vi "ExSubSetPulserInSpeFileHeader.vi"(3 "error in (no error)":errorcluster, 4 "Pulser Handle":u32, 5 "File Handle":u32) -> (0 "error out":errorcluster, 1 "Pulser Handle":u32, 2 "File Handle":u32)   [LabVIEW 2010]
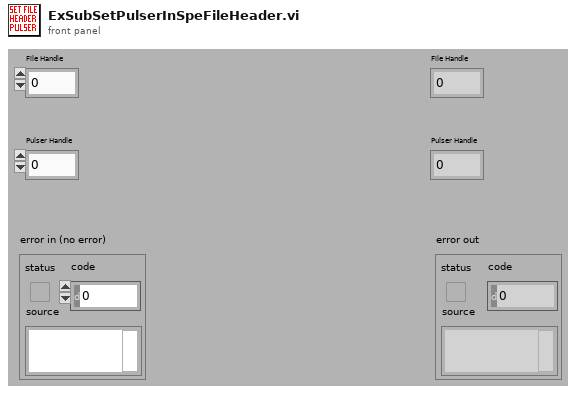
[diagram p1: front panel]
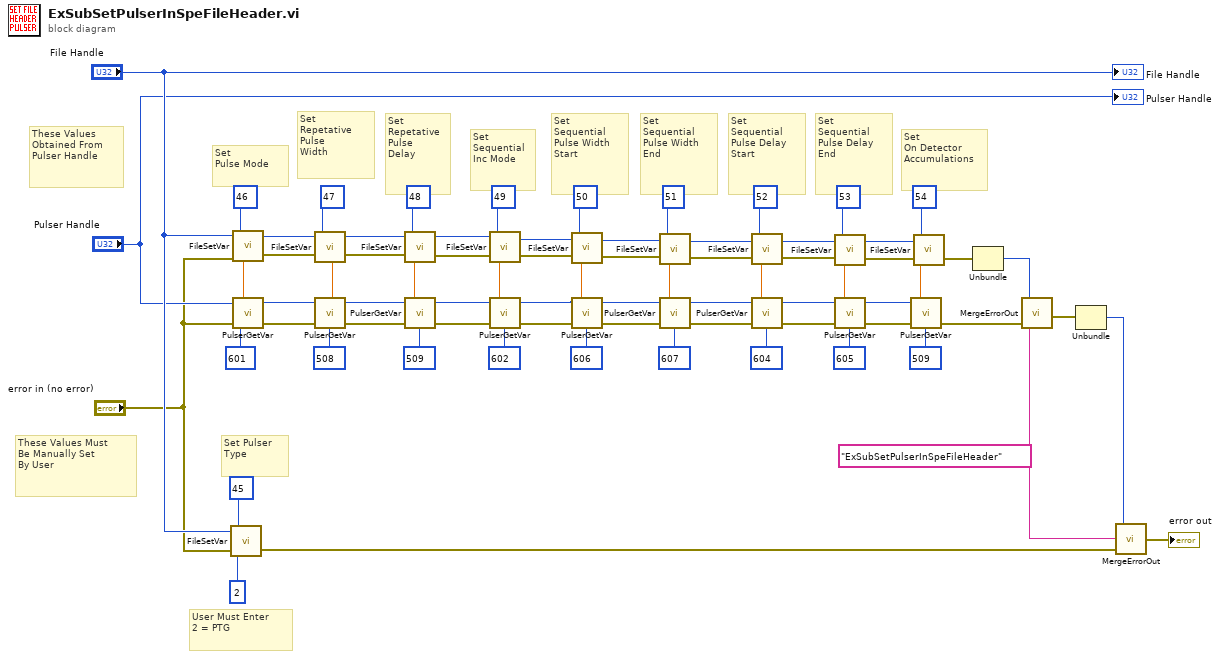
[diagram p0: block diagram]
diagram:
  w7 = "ExSubSetPulserInSpeFileHeader"
  # "These Values Must\nBe Manually Set\nBy User"
  # "These Values\nObtained From\nPulser Handle"
  # "User Must Enter\n2 = PTG"
  # "Set Pulser\nType"
  # "Set \nOn Detector\nAccumulations"
  # "Set\nSequential\nPulse Delay\nEnd"
  # "Set\nSequential\nPulse Delay\nStart"
  # "Set\nSequential\nPulse Width\nEnd"
  # "Set\nSequential\nPulse Width\nStart"
  # "Set\nSequential\nInc Mode"
  # "Set\nRepetative\nPulse\nDelay"
  # "Set\nRepetative\nPulse\nWidth"
  # "Set\nPulse Mode"
  n1 = call <userlib>:"FileSetVar.vi"("error in"="error in (no error)", "Value"=2, "Parameter ID"=45, "File Handle"="File Handle") -> ("error out"=w3:errorcluster)  [unwired: 1 out]
  n2 = call <userlib>:"PulserGetVar.vi"("error in (no error)"="error in (no error)", "Parameter ID"=601, "Pulser Handle"="Pulser Handle") -> ("error out"=w60:errorcluster, "Value"=w70:dbl, "Pulser Handle"=w62:u32)
  n3 = call <userlib>:"FileSetVar.vi"("error in"="error in (no error)", "Value"=w70, "Parameter ID"=46, "File Handle"="File Handle") -> ("error out"=w58:errorcluster, "File Handle"=w67:u32)
  n4 = call <userlib>:"PulserGetVar.vi"("error in (no error)"=w60, "Parameter ID"=508, "Pulser Handle"=w62) -> ("error out"=w59:errorcluster, "Value"=w57:dbl, "Pulser Handle"=w61:u32)
  n5 = call <userlib>:"FileSetVar.vi"("error in"=w58, "Value"=w57, "Parameter ID"=47, "File Handle"=w67) -> ("error out"=w65:errorcluster, "File Handle"=w66:u32)
  n6 = call <userlib>:"PulserGetVar.vi"("error in (no error)"=w59, "Parameter ID"=509, "Pulser Handle"=w61) -> ("error out"=w49:errorcluster, "Value"=w56:dbl, "Pulser Handle"=w50:u32)
  n7 = call <userlib>:"FileSetVar.vi"("error in"=w65, "Value"=w56, "Parameter ID"=48, "File Handle"=w66) -> ("error out"=w51:errorcluster, "File Handle"=w52:u32)
  n8 = call <userlib>:"PulserGetVar.vi"("error in (no error)"=w49, "Parameter ID"=602, "Pulser Handle"=w50) -> ("error out"=w24:errorcluster, "Value"=w53:dbl, "Pulser Handle"=w28:u32)
  n9 = call <userlib>:"FileSetVar.vi"("error in"=w51, "Value"=w53, "Parameter ID"=49, "File Handle"=w52) -> ("error out"=w32:errorcluster, "File Handle"=w36:u32)
  n10 = call <userlib>:"PulserGetVar.vi"("error in (no error)"=w24, "Parameter ID"=606, "Pulser Handle"=w28) -> ("error out"=w23:errorcluster, "Value"=w46:dbl, "Pulser Handle"=w27:u32)
  n11 = call <userlib>:"FileSetVar.vi"("error in"=w32, "Value"=w46, "Parameter ID"=50, "File Handle"=w36) -> ("error out"=w31:errorcluster, "File Handle"=w35:u32)
  n12 = call <userlib>:"PulserGetVar.vi"("error in (no error)"=w23, "Parameter ID"=607, "Pulser Handle"=w27) -> ("error out"=w22:errorcluster, "Value"=w43:dbl, "Pulser Handle"=w26:u32)
  n13 = call <userlib>:"FileSetVar.vi"("error in"=w31, "Value"=w43, "Parameter ID"=51, "File Handle"=w35) -> ("error out"=w30:errorcluster, "File Handle"=w34:u32)
  n14 = call <userlib>:"PulserGetVar.vi"("error in (no error)"=w22, "Parameter ID"=604, "Pulser Handle"=w26) -> ("error out"=w21:errorcluster, "Value"=w40:dbl, "Pulser Handle"=w25:u32)
  n15 = call <userlib>:"FileSetVar.vi"("error in"=w30, "Value"=w40, "Parameter ID"=52, "File Handle"=w34) -> ("error out"=w29:errorcluster, "File Handle"=w33:u32)
  n16 = call <userlib>:"PulserGetVar.vi"("error in (no error)"=w21, "Parameter ID"=605, "Pulser Handle"=w25) -> ("error out"=w14:errorcluster, "Value"=w37:dbl, "Pulser Handle"=w15:u32)
  n17 = call <userlib>:"FileSetVar.vi"("error in"=w29, "Value"=w37, "Parameter ID"=53, "File Handle"=w33) -> ("error out"=w16:errorcluster, "File Handle"=w17:u32)
  n18 = call <userlib>:"PulserGetVar.vi"("error in (no error)"=w14, "Parameter ID"=509, "Pulser Handle"=w15) -> ("error out"=w1:errorcluster, "Value"=w18:dbl)  [unwired: 1 out]
  n19 = call <userlib>:"FileSetVar.vi"("error in"=w16, "Value"=w18, "Parameter ID"=54, "File Handle"=w17) -> ("error out"=w2:errorcluster)  [unwired: 1 out]
  n20 = Unbundle(w2) -> ("code"=w10:i32)  [unwired: 2 out]
  n21 = call <userlib>:"MergeErrorOut.vi"("error in"=w1, "Fucntion Name"=w7, "ErrorCode"=w10) -> ("error out"=w4:errorcluster)
  n22 = Unbundle(w4) -> ("code"=w8:i32)  [unwired: 2 out]
  n23 = call <userlib>:"MergeErrorOut.vi"("error in"=w3, "Fucntion Name"=w7, "ErrorCode"=w8) -> ("error out"=→"error out":errorcluster)
  "File Handle" <- "File Handle"
  "Pulser Handle" <- "Pulser Handle"
